vi "前序状态.vi"(10 "前序设备编号":string, 11 "前序追溯码":string) -> (3 "前序状态":string)   [LabVIEW 2020]
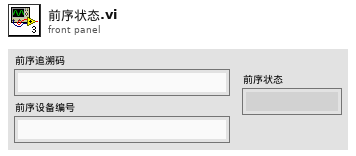
[diagram p1: front panel]
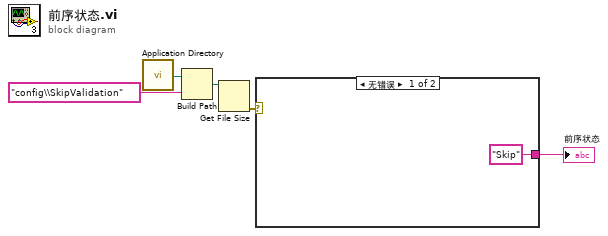
[diagram p0: block diagram]
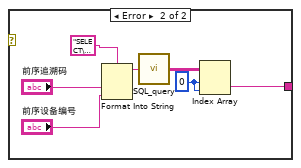
[diagram p2: hidden frame]
diagram:
  n1 = call <vilib>:"Application Directory.vi"() -> ("Application Directory"=w5:path)
  n2 = Build Path(base path=w5, name or relative path="config\\SkipValidation" ("名称或相对路径")) -> (appended path=w3:path)
  n3 = Get File Size(file=w3) -> (0:w2:errorcluster)  [unwired: 1 in, 2 out]
  n4 = case shown="无错误" w2 {
    tunnel: ["Skip" w7] -> w1
    frame No Error {
    }
    frame Error {
      w10 = 0 ("索引 (行)")
      n5 = Format Into String(format string="SELECT\n\tdbo.[产品质量1].[加工状态]\nFROM\n\tdbo.[产品质量1]\nWHERE\n\tdbo.[产品质量1].[工位追溯码] = '%s'\nAND dbo.[产品质量1].[设备编号] = '%s'\n", "前序追溯码", "前序设备编号") -> (resulting string=w12:string)  [unwired: 2 in, 1 out]
      n6 = call "SQL_query.vi"("SQL query"=w12) -> ("data"=w11:string[][])  [unwired: 2 in, 2 out]
      n7 = Index Array(array=w11, index (row)=w10, index (col)=w10) -> (element=w7:string)
    }
  }
  "前序状态" <- w1
